vi "get AdjacentMines.vi"(8 "error in (no error)":errorcluster, 11 "Cell in":refnum<class "Cell.lvclass">) -> (0 "error out":errorcluster, 1 "hasFlag":bool, 2 "isCovered":bool, 3 "AdjacentMines":dbl)   [LabVIEW 2014, in "Cell.lvclass"]
uses:
  Cell.lvclass
  Cell.lvclass/Cell.ctl
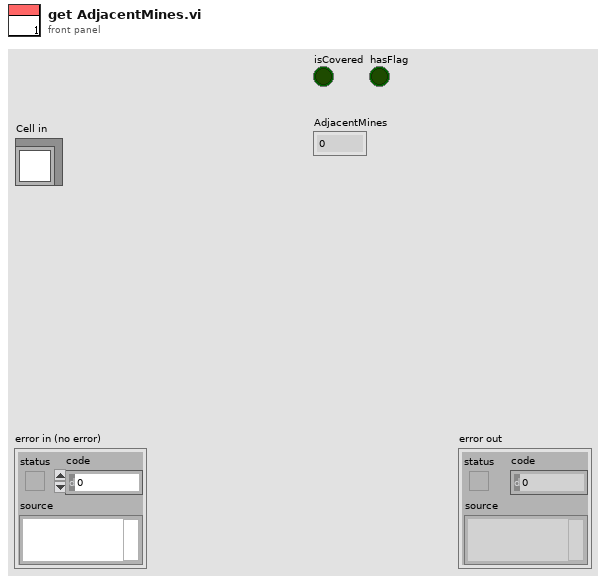
[diagram p1: front panel]
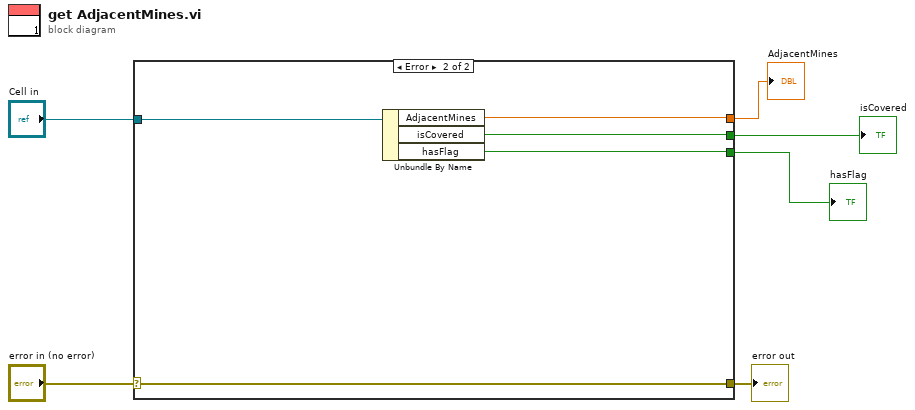
[diagram p0: block diagram]
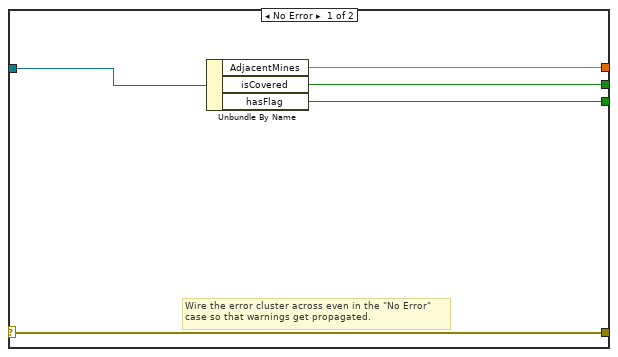
[diagram p2: hidden frame]
diagram:
  n1 = case shown="Error" "error in (no error)" {
    selector: "error in (no error)" -> [w11 w16]
    tunnel: [w11 w16] -> w5
    tunnel: "Cell in" -> [w10 w15]
    tunnel: [w9 w14] -> w3
    tunnel: [w8 w13] -> w2
    tunnel: [w7 w12] -> w1
    frame No Error {
      # "Wire the error cluster across even in the \"No Error\"\ncase so that warnings get propagated."
      n2 = Unbundle By Name(w10) -> ("AdjacentMines"=w9:dbl, "isCovered"=w8:bool, "hasFlag"=w7:bool)
    }
    frame Error {
      n3 = Unbundle By Name(w15) -> ("AdjacentMines"=w14:dbl, "isCovered"=w13:bool, "hasFlag"=w12:bool)
    }
  }
  "error out" <- w5
  "AdjacentMines" <- w3
  "isCovered" <- w2
  "hasFlag" <- w1
